vi "Accurate Measure With Setting.vi"(0 "DMM ref in":refnum<visa-resource-name>, 1 "Accurate Measure Setting":T1={"Enable DMM Relay"=FALSE, "Measure Current Only"=FALSE, [], "channel_count"=11}, 2 "P_current_count":i32, 3 "N_current_count":i32, 5 "DMM error in":errorcluster, 7 "Current Sense \nResitance Array":dbl[](array[numeric])=[1.0032214, 1.00250644, 1.00234822, 1.0040944, 1.0017711, 1.00229431, 1.00344206, 1.00482066, 1.00381056, 1.00290978, 1.00333016, 1.00367587], 9 "ESP32 ref in":refnum<visa-resource-name>, 11 "ESP32 error in":errorcluster, 12 "current_mode":u8[](array[numeric])=[0, 0, 0, 0, 0, 0, 0, 0, 0, 0, 0]) -> (4 "DMM ref out":refnum<visa-resource-name>, 6 "DMM error out":errorcluster, 8 "Accurate Data":dbl[](array[numeric]), 10 "ESP32 ref out":refnum<visa-resource-name>, 13 "time_out_count":i32, 14 "Standard Deviation of Data":dbl[](array[numeric]), 15 "ESP32 error out":errorcluster)   [LabVIEW 2023]
uses:
  <instrlib>/Agilent 3446X Series/Agilent 3446X Series.lvlib
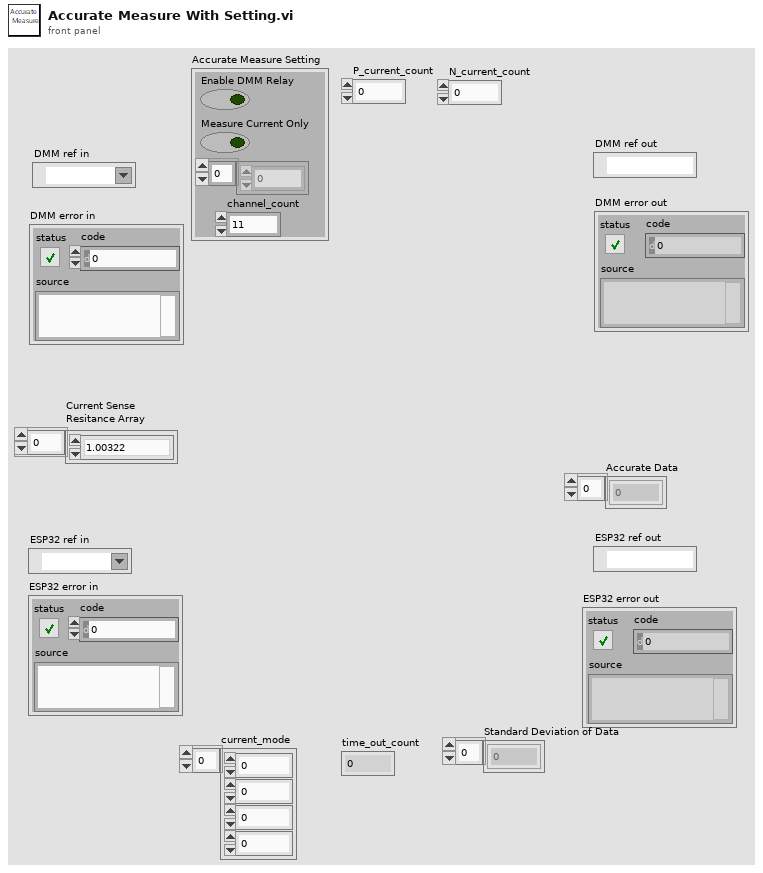
[diagram p1: front panel]
types:
  T1 = cluster{"Enable DMM Relay":bool, "Measure Current Only":bool, dbl[], "channel_count":i32}
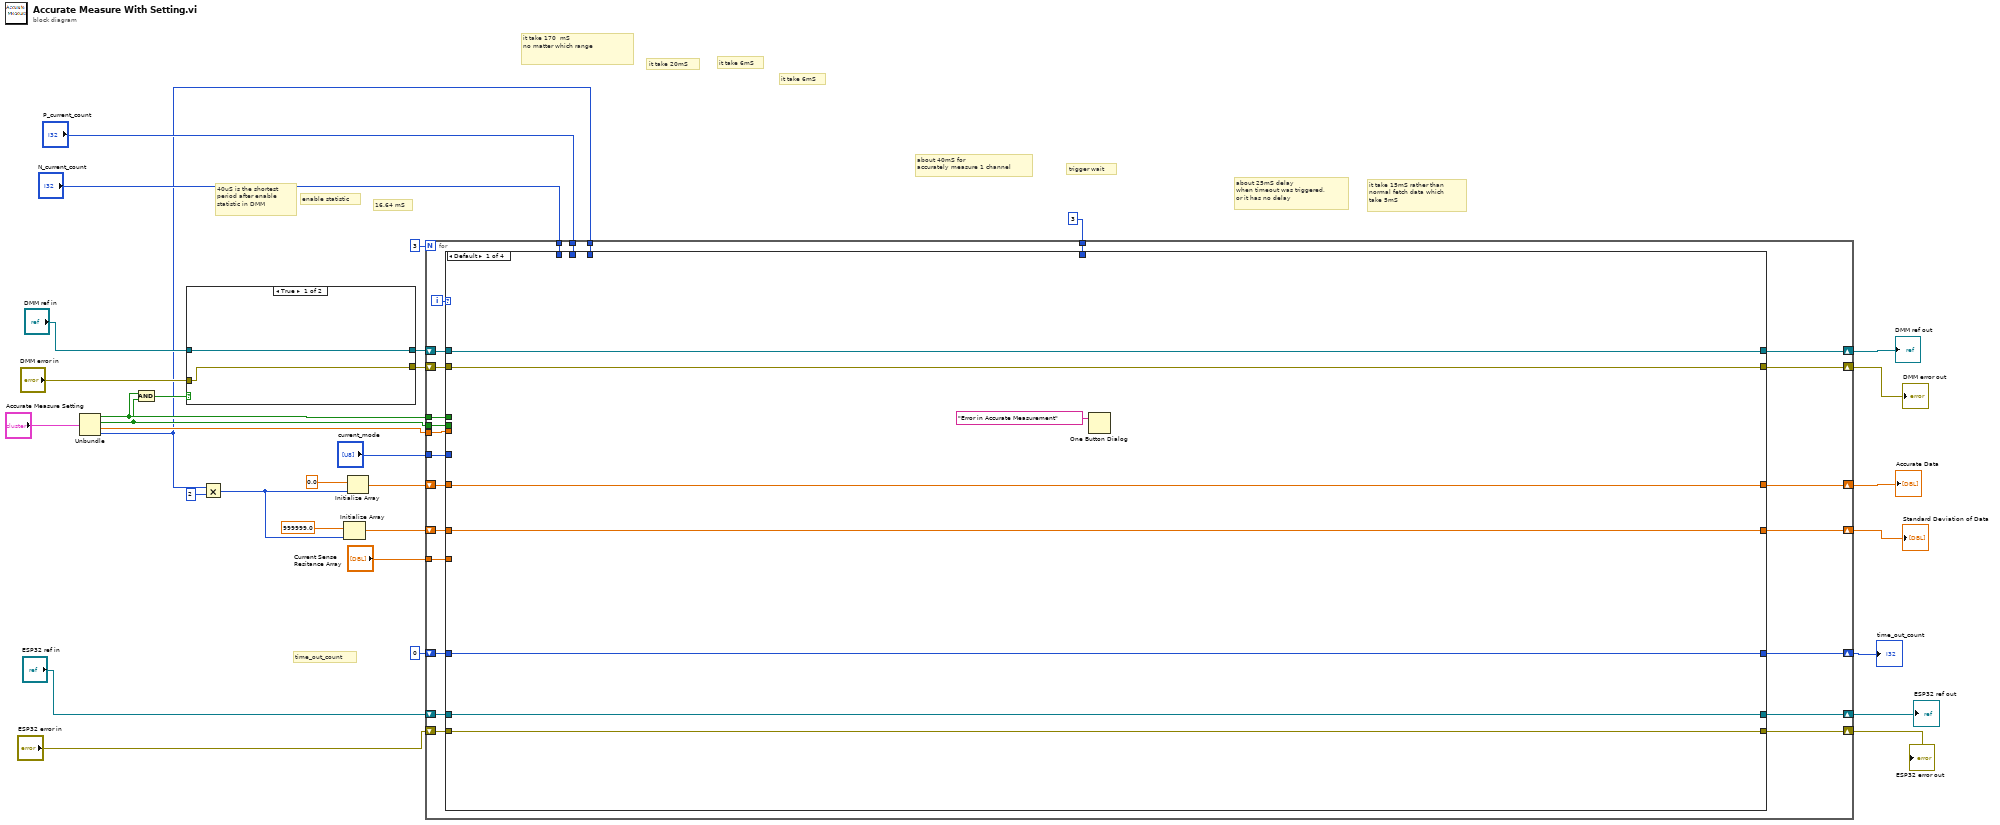
[diagram p0: block diagram]
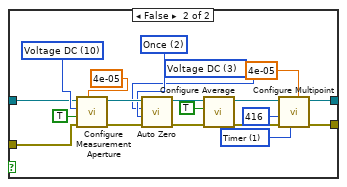
[diagram p2: hidden frame]
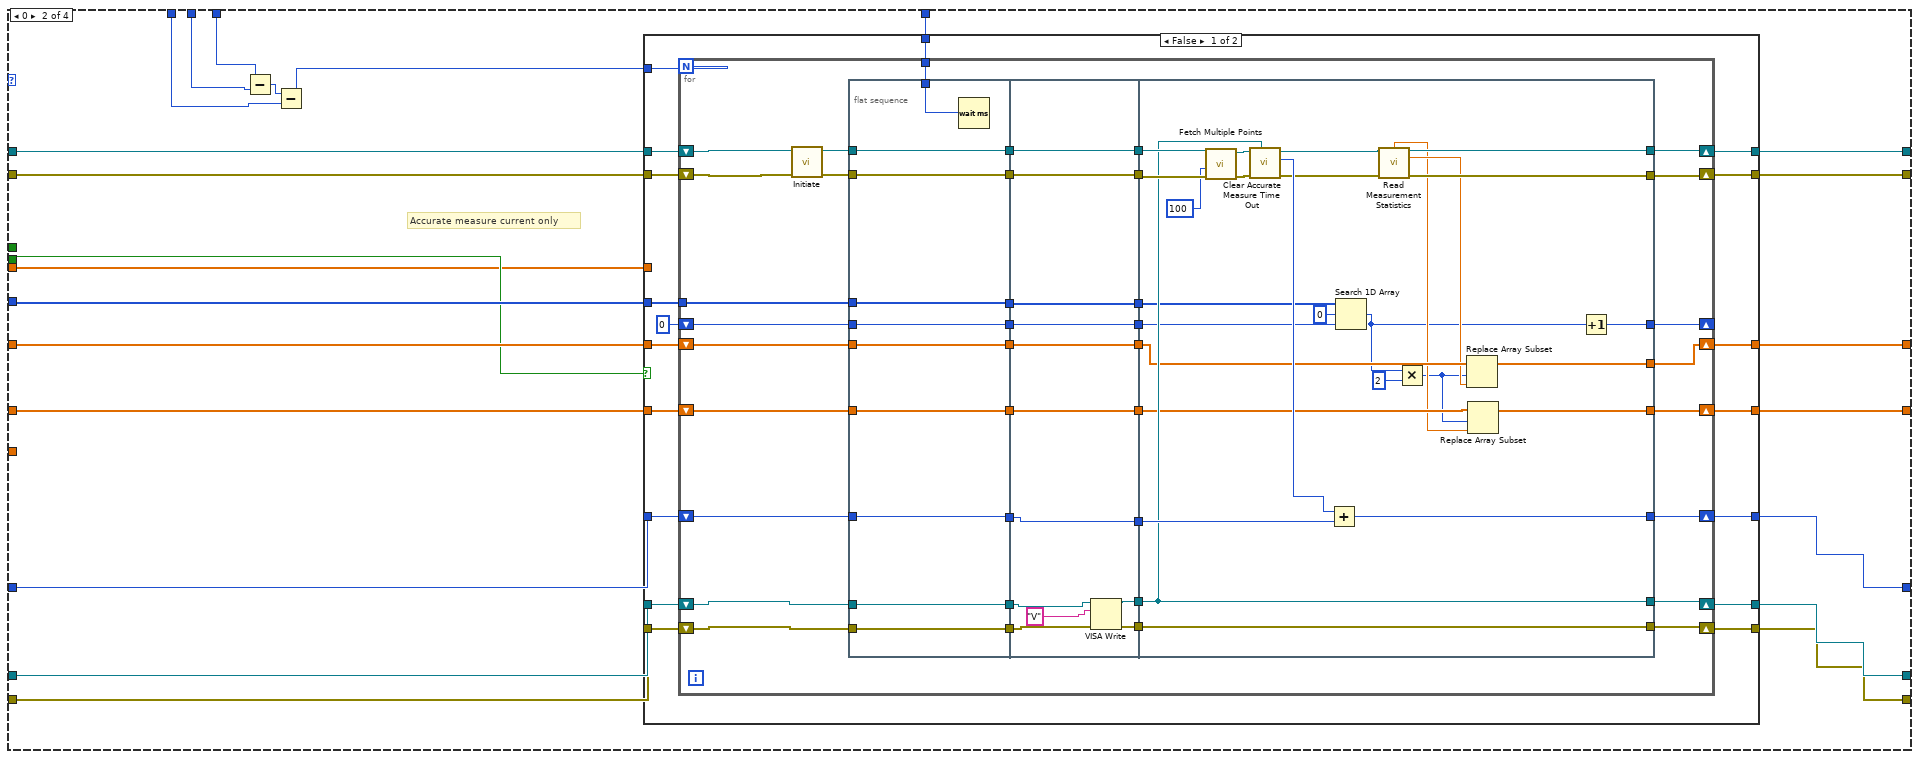
[diagram p3: hidden frame]
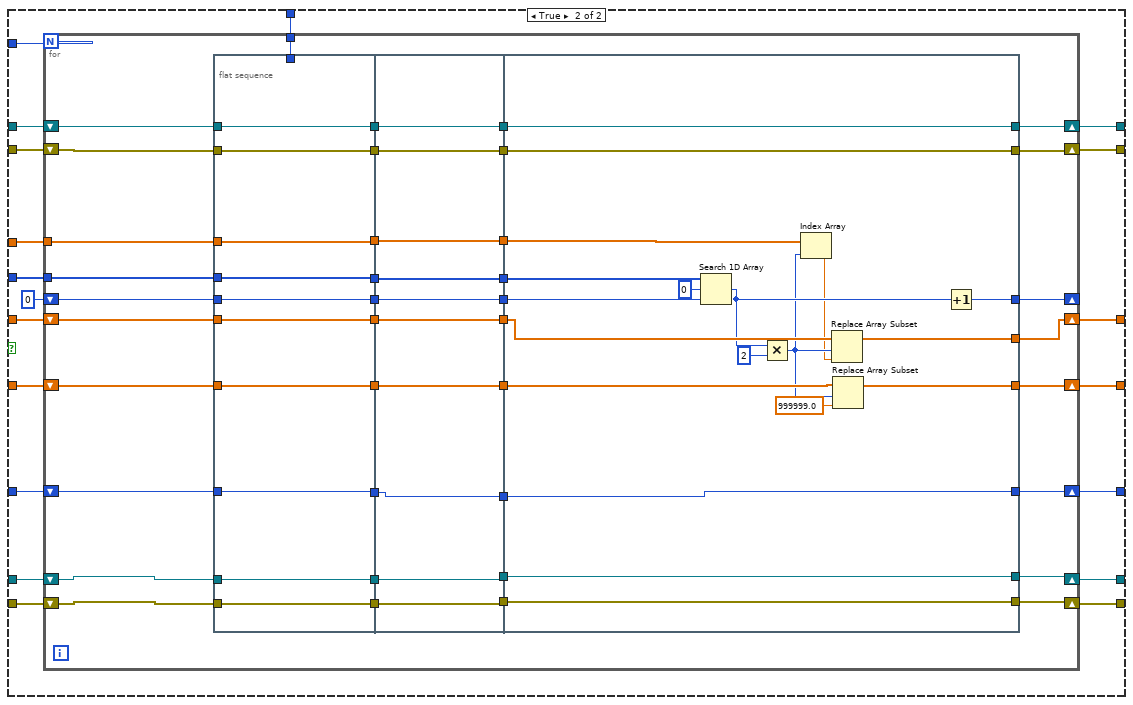
[diagram p4: hidden frame]
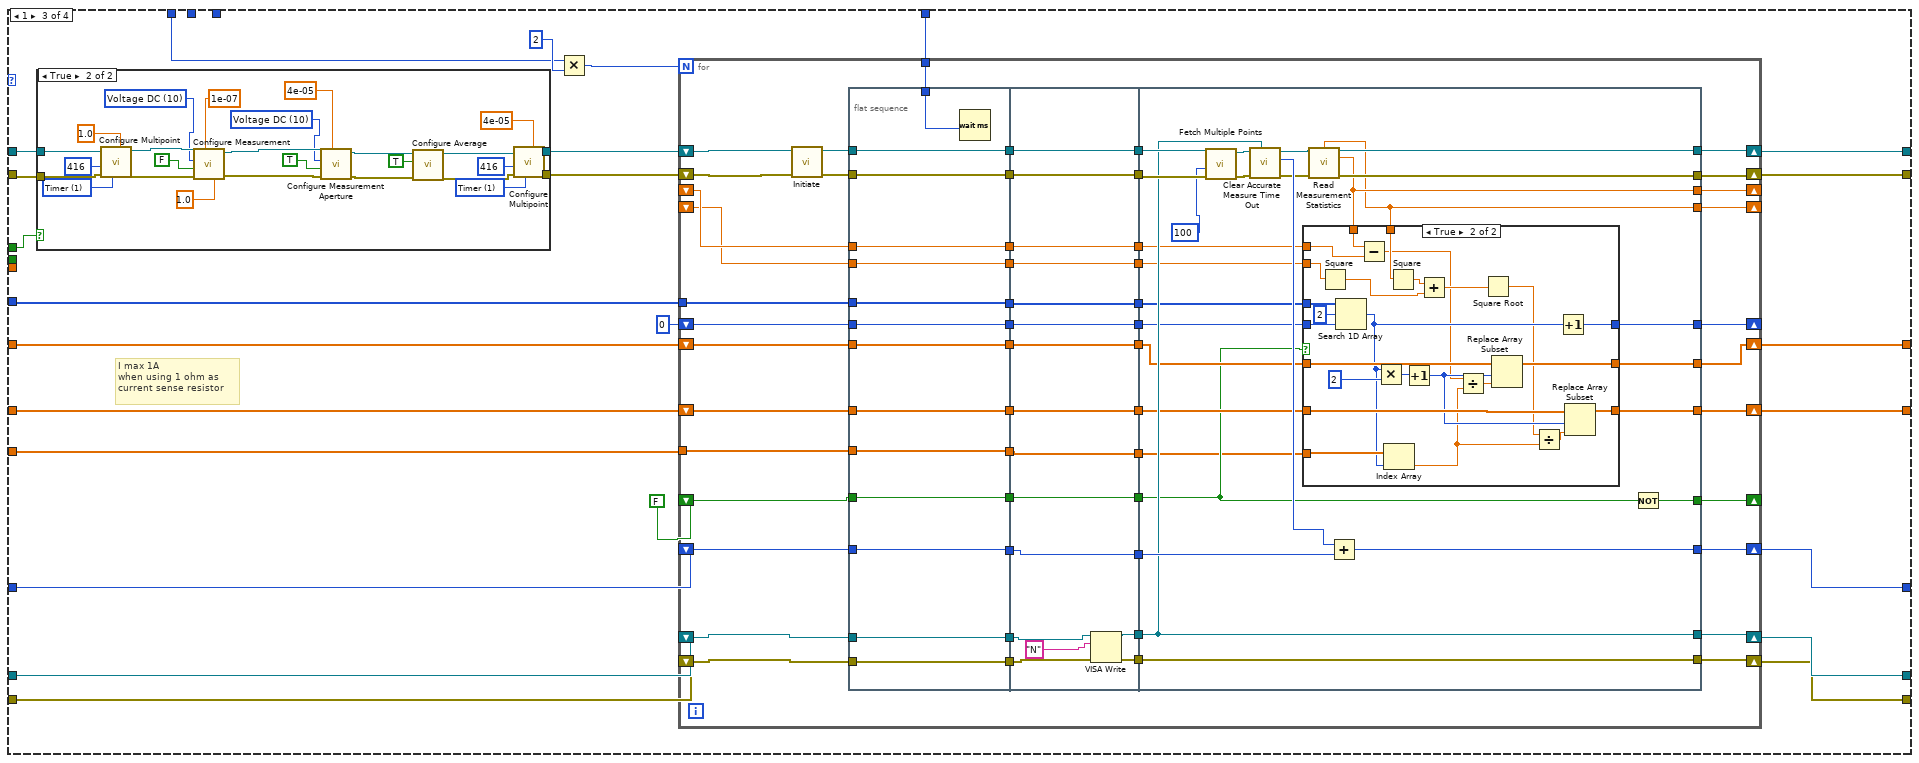
[diagram p5: hidden frame]
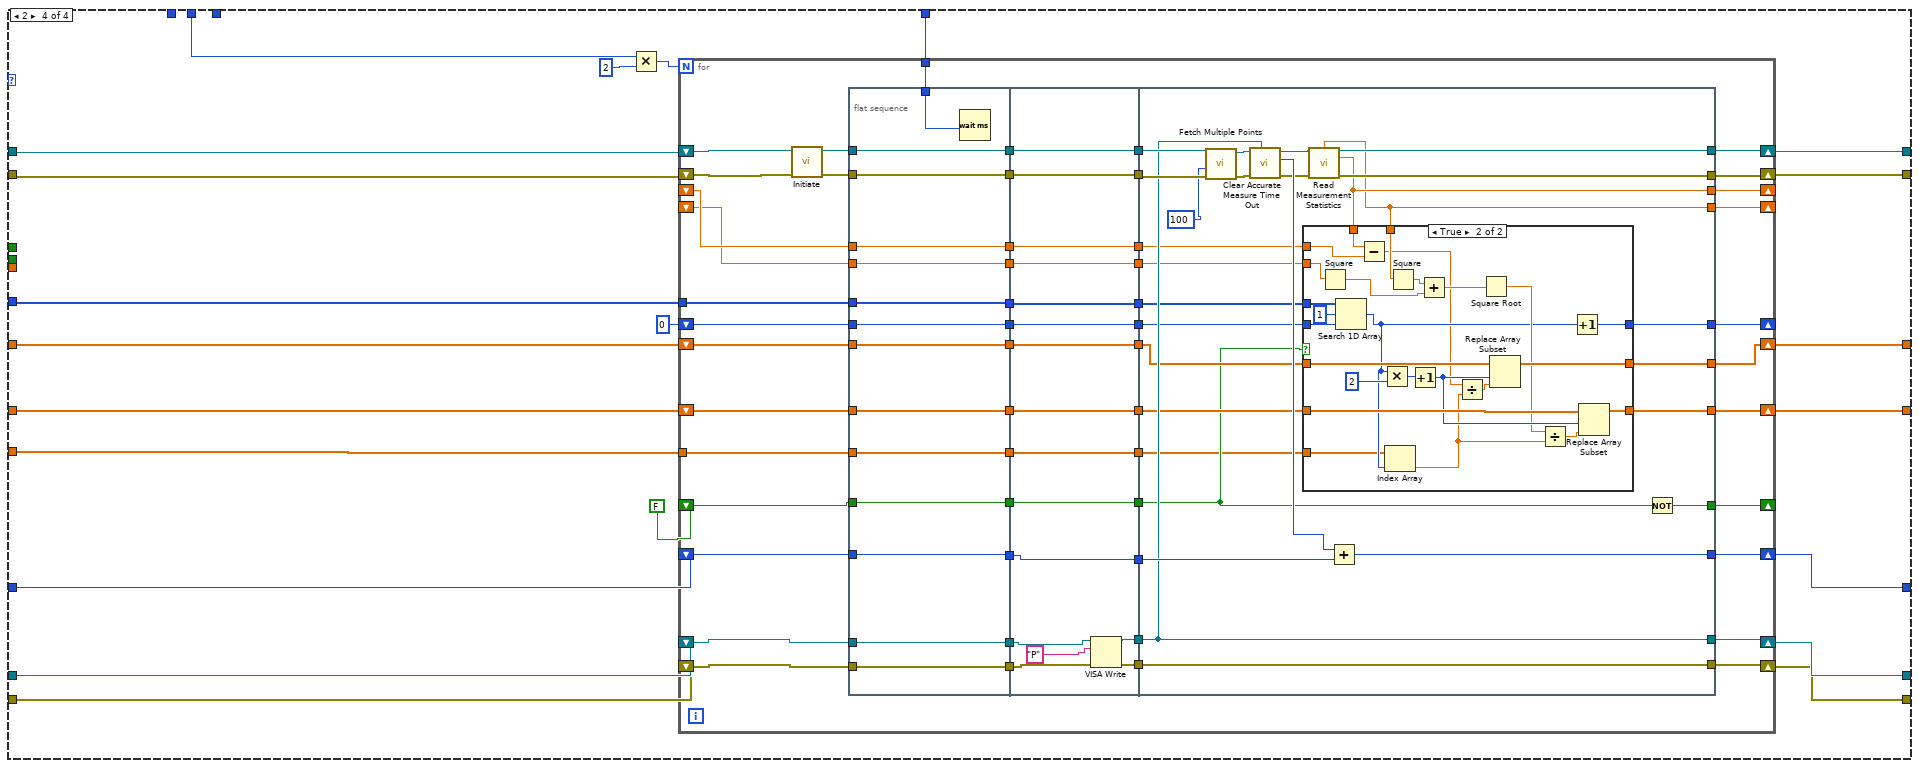
[diagram p8: hidden frame]
diagram:
  # "it take 6mS"
  # "it take 6mS"
  # "it take 20mS"
  # "it take 170  mS\nno matter which range"
  # "it take 15mS rather than\nnormal fetch data which \ntake 5mS"
  # "about 40mS for \naccurately measure 1 channel"
  # "about 25mS delay\nwhen timeout was triggered,\nor it has no delay"
  # "time_out_count"
  # "trigger wait"
  # "16.64 mS"
  # "enable statistic"
  # "40uS is the shortest\nperiod after enable \nstatistic in DMM"
  n1 = Unbundle("Accurate Measure Setting") -> ("Enable DMM Relay"=w5:bool, "Measure Current Only"=w4:bool, w6:dbl[], "channel_count"=w2:i32)
  n2 = And(x=w5, y=w4) -> (x .and. y?=w3:bool)
  n3 = case shown="True" w3 {
    tunnel: [w34 w38] -> w32
    tunnel: [w33 w37] -> w31
    tunnel: "DMM ref in" -> [w34 w36]
    tunnel: "DMM error in" -> [w33 w35]
    frame True {
    }
    frame False {
      w40 = 1 items=["Immediate", "Timer"] ("Sample Source (0: Immediate)")
      w47 = 3 items=["Current DC", "Resistance", "Temperature", "Voltage DC"] ("Zero Type (0: Current DC)")
      w48 = 2 items=["Disable", "Enable", "Once"] ("Auto Zero (1: Enable)")
      w44 = 10 items=["Continuity", "Current AC", "Current DC", "Diode", "Frequency", "Resistance 4-wire", "Period", "Resistance 2-wire", "Temperature", "Voltage AC", "Voltage DC", "Voltage DC Ratio", "Capacitance"] ("Measurement Function (0: Continuity)")
      n4 = call <instrlib>:"Configure Measurement Aperture.vi"("Aperture Time (0.1s)"=4e-05, "error in (no error)"=w35, "Enable Aperture (F: Disable)"=TRUE, "Measurement Function (0: Continuity)"=w44, "VISA resource name"=w36) -> ("error out"=w51:errorcluster, "VISA resource name out"=w50:refnum<visa-resource-name>)  [unwired: 5 in]
      n5 = call <instrlib>:"Auto Zero.vi"("error in (no error)"=w51, "Auto Zero (1: Enable)"=w48, "Zero Type (0: Current DC)"=w47, "VISA resource name"=w50) -> ("error out"=w53:errorcluster, "VISA resource name out"=w52:refnum<visa-resource-name>)  [unwired: 6 in]
      n6 = call <instrlib>:"Configure Average.vi"("error in (no error)"=w53, "Enable Statistics (F: Disable)"=TRUE, "VISA resource name"=w52) -> ("error out"=w42:errorcluster, "VISA resource name out"=w43:refnum<visa-resource-name>)  [unwired: 7 in]
      n7 = call <instrlib>:"Configure Multipoint.vi"("Sample Interval (1 Second)"=4e-05, "Sample Source (0: Immediate)"=w40, "error in (no error)"=w42, "Sample Count (1)"=416, "VISA resource name"=w43) -> ("error out"=w37:errorcluster, "VISA resource name out"=w38:refnum<visa-resource-name>)  [unwired: 2 in, 3 out]
    }
  }
  n8 = Multiply(x=w2, y=2) -> (x*y=w8:i32)
  n9 = Initialize Array(999999.0 ("Arithmetic Mean"), w8) -> (w17:dbl[])
  n10 = Initialize Array(0.0 ("Arithmetic Mean"), w8) -> (w20:dbl[])
  n11 = for {
    N: 3 -> [_]
    shift-right: [w75] -> w13
    shift-left: "ESP32 ref in" -> [w77]
    shift-right: [w74] -> w12
    shift-left: "ESP32 error in" -> [w76]
    shift-right: [w71] -> w15
    shift-left: w32 -> [w73]
    shift-right: [w70] -> w14
    shift-left: w31 -> [w72]
    tunnel: w2 -> [w69]
    tunnel: "P_current_count" -> [w68]
    tunnel: "N_current_count" -> [w67]
    tunnel: u32 3 ("milliseconds to wait") -> [w66]
    shift-right: [w65] -> w22
    shift-left: 0 -> [w64]
    shift-right: [w58] -> w11
    shift-left: w20 -> [w63]
    tunnel: "current_mode" -> [w62]
    shift-right: [w59] -> w10
    shift-left: w17 -> [w60]
    tunnel: w5 -> [w57]
    tunnel: w4 -> [w56]
    tunnel: w6 -> [w55]
    tunnel: "Current Sense \nResitance Array" -> [w54]
    i -> [w61]
    n12 = case shown="Default" w61 {
      tunnel: w77 -> [w83 w104 w335 w524]
      tunnel: w76 -> [w82 w103 w334 w523]
      tunnel: [w83 w100 w331 w520] -> w75
      tunnel: [w82 w99 w330 w519] -> w74
      tunnel: w73 -> [w85 w106 w319 w505]
      tunnel: w72 -> [w84 w105 w318 w504]
      tunnel: [w85 w102 w333 w522] -> w71
      tunnel: [w84 w101 w332 w521] -> w70
      tunnel: w69 -> [_ w98 _ _]
      tunnel: w68 -> [_ w97 _ w507]
      tunnel: w67 -> [_ w96 w314 _]
      tunnel: [w79 w94 w328 w517] -> w65
      tunnel: w66 -> [_ w95 w329 w518]
      tunnel: w64 -> [w79 w93 w327 w516]
      tunnel: w63 -> [w81 w91 w325 w514]
      tunnel: w62 -> [_ w92 w326 w515]
      tunnel: w60 -> [w80 w90 w323 w512]
      tunnel: [w80 w89 w322 w511] -> w59
      tunnel: [w81 w88 w321 w510] -> w58
      tunnel: w57 -> [_ _ w312 _]
      tunnel: w56 -> [_ w87 _ _]
      tunnel: w55 -> [_ w86 _ _]
      tunnel: w54 -> [_ _ w311 w503]
      frame Default {
        n13 = One Button Dialog(message="Error in Accurate Measurement") -> ()  [unwired: 1 in, 1 out]
      }
      frame 0 {
        # "Accurate measure current only"
        n14 = Subtract(x=w98, y=w97) -> (x-y=w108:i32)
        n15 = Subtract(x=w108, y=w96) -> (x-y=w107:i32)
        n16 = case shown="False" w87 {
          tunnel: w107 -> [w126 w232]
          tunnel: w106 -> [w125 w231]
          tunnel: w105 -> [w124 w230]
          tunnel: w104 -> [w123 w229]
          tunnel: w103 -> [w122 w228]
          tunnel: [w121 w227] -> w102
          tunnel: [w120 w226] -> w101
          tunnel: [w119 w225] -> w100
          tunnel: [w118 w224] -> w99
          tunnel: w95 -> [w117 w223]
          tunnel: [w116 w222] -> w94
          tunnel: w93 -> [w115 w221]
          tunnel: w92 -> [w114 w220]
          tunnel: w91 -> [w113 w219]
          tunnel: w90 -> [w111 w217]
          tunnel: [w110 w216] -> w89
          tunnel: [w109 w215] -> w88
          tunnel: w86 -> [_ w214]
          frame False {
            n17 = for {
              N: w126 -> [_]
              shift-right: [w160] -> w121
              shift-left: w125 -> [w164]
              shift-right: [w159] -> w120
              shift-left: w124 -> [w163]
              shift-right: [w158] -> w119
              shift-left: w123 -> [w162]
              shift-right: [w157] -> w118
              shift-left: w122 -> [w161]
              tunnel: w117 -> [w143]
              shift-right: [w142] -> w116
              shift-left: w115 -> [w156]
              tunnel: w114 -> [w140]
              shift-right: [w128] -> w109
              shift-left: w113 -> [w137]
              shift-right: [w132] -> _
              shift-left: 0 ("index of element") -> [w133]
              shift-right: [w127] -> w110
              shift-left: w111 -> [w130]
              n18 = call <instrlib>:"Initiate.vi"("error in (no error)"=w163, "VISA resource name"=w164) -> ("error out"=w144:errorcluster, "VISA resource name out"=w145:refnum<visa-resource-name>)  [unwired: 8 in]
              n19 = flat-sequence {
                tunnel: [w174] -> w155
                tunnel: w162 -> [w174]
                tunnel: [w173] -> w154
                tunnel: w161 -> [w173]
                tunnel: w145 -> [w172]
                tunnel: [w172] -> w153
                tunnel: [w171] -> w152
                tunnel: w144 -> [w171]
                tunnel: [w170] -> w151
                tunnel: w156 -> [w170]
                tunnel: w143 -> [w169]
                tunnel: [w168] -> w141
                tunnel: w140 -> [w168]
                tunnel: [w167] -> w138
                tunnel: w137 -> [w167]
                tunnel: w133 -> [w166]
                tunnel: [w166] -> w135
                tunnel: [w165] -> w131
                tunnel: w130 -> [w165]
                tunnel: w155 -> [w186]
                tunnel: w154 -> [w185]
                tunnel: w153 -> [w184]
                tunnel: [w184] -> w147
                tunnel: w152 -> [w183]
                tunnel: [w183] -> w148
                tunnel: [w182] -> w149
                tunnel: [w181] -> w150
                tunnel: w151 -> [w179]
                tunnel: [w179] -> w146
                tunnel: w141 -> [w178]
                tunnel: [w178] -> w139
                tunnel: w138 -> [w177]
                tunnel: [w177] -> w136
                tunnel: w135 -> [w176]
                tunnel: [w176] -> w134
                tunnel: w131 -> [w175]
                tunnel: [w175] -> w129
                tunnel: [w213] -> w157
                tunnel: [w201] -> w158
                tunnel: [w205] -> w159
                tunnel: [w206] -> w160
                tunnel: w150 -> [w213]
                tunnel: w149 -> [w201]
                tunnel: w148 -> [w212]
                tunnel: w147 -> [w211]
                tunnel: [w207] -> w142
                tunnel: w146 -> [w202]
                tunnel: w139 -> [w200]
                tunnel: w136 -> [w196]
                tunnel: w134 -> [w198]
                tunnel: [w197] -> w132
                tunnel: w129 -> [w194]
                tunnel: [w192] -> w128
                tunnel: [w191] -> w127
                frame #0 {
                  n20 = Wait (ms)(milliseconds to wait=w169) -> ()  [unwired: 1 out]
                }
                frame #1 {
                  n21 = VISA Write(VISA resource name=w186, write buffer="V" ("data in"), error in (no error)=w185) -> (VISA resource name out=w182:refnum<visa-resource-name>, error out=w181:errorcluster)  [unwired: 1 out]
                }
                frame #2 {
                  n22 = call <instrlib>:"Fetch Multiple Points.vi"("error in (no error)"=w212, "Timeout (10000 ms)"=100, "VISA resource name"=w211) -> ("error out"=w209:errorcluster, "VISA resource name out"=w210:refnum<visa-resource-name>)  [unwired: 1 in, 6 out]
                  n23 = call "Clear Accurate Measure Time Out.vi"("ESP32 ref"=w201, "error in (no error)"=w209, "DMM ref"=w210) -> ("error out"=w203:errorcluster, "Time out count"=w208:i32, "VISA Refnum out"=w204:refnum<visa-resource-name>)  [unwired: 5 in, 1 out]
                  n24 = Add(x=w208, y=w202) -> (x+y=w207:i32)
                  n25 = Search 1D Array(1D array=w200, element=u8 0, start index (0)=w198) -> (index of element=w189:i32)
                  n26 = call <instrlib>:"Read Measurement Statistics.vi"("VISA resource name"=w204, "error in (no error)"=w203) -> ("Standard Deviation"=w193:dbl, "VISA resource name out"=w206:refnum<visa-resource-name>, "Arithmetic Mean"=w195:dbl, "error out"=w205:errorcluster)  [unwired: 6 in, 4 out]
                  n27 = Multiply(x=w189, y=2) -> (x*y=w187:i32)
                  n28 = Replace Array Subset(array=w196, new element=w195, index=w187) -> (w192:dbl[])
                  n29 = Replace Array Subset(array=w194, new element=w193, index=w187) -> (w191:dbl[])
                  n30 = Increment(x=w189) -> (x+1=w197:i32)
                }
              }
            }
          }
          frame True {
            n31 = for {
              N: w232 -> [_]
              shift-right: [w241] -> w227
              shift-left: w231 -> [w243]
              shift-right: [w236] -> w226
              shift-left: w230 -> [w238]
              shift-right: [w269] -> w225
              shift-left: w229 -> [w271]
              shift-right: [w268] -> w224
              shift-left: w228 -> [w270]
              tunnel: w223 -> [w260]
              shift-right: [w259] -> w222
              shift-left: w221 -> [w267]
              tunnel: w220 -> [w257]
              shift-right: [w245] -> w215
              shift-left: w219 -> [w254]
              shift-right: [w249] -> _
              shift-left: 0 ("index of element") -> [w250]
              shift-right: [w244] -> w216
              shift-left: w217 -> [w247]
              tunnel: w214 -> [w233]
              n32 = flat-sequence {
                tunnel: [w281] -> w266
                tunnel: w271 -> [w281]
                tunnel: [w280] -> w265
                tunnel: w270 -> [w280]
                tunnel: [w279] -> w264
                tunnel: w267 -> [w279]
                tunnel: w260 -> [_]
                tunnel: [w278] -> w258
                tunnel: w257 -> [w278]
                tunnel: [w277] -> w255
                tunnel: w254 -> [w277]
                tunnel: w250 -> [w276]
                tunnel: [w276] -> w252
                tunnel: [w275] -> w248
                tunnel: w247 -> [w275]
                tunnel: w243 -> [w274]
                tunnel: [w274] -> w240
                tunnel: [w273] -> w239
                tunnel: w238 -> [w273]
                tunnel: [w272] -> w235
                tunnel: w233 -> [w272]
                tunnel: w266 -> [w284]
                tunnel: w265 -> [w283]
                tunnel: [w284] -> w262
                tunnel: [w283] -> w263
                tunnel: w264 -> [w291]
                tunnel: [w291] -> w261
                tunnel: w258 -> [w290]
                tunnel: [w290] -> w256
                tunnel: w255 -> [w289]
                tunnel: [w289] -> w253
                tunnel: w252 -> [w288]
                tunnel: [w288] -> w251
                tunnel: w248 -> [w287]
                tunnel: [w287] -> w246
                tunnel: [w286] -> w242
                tunnel: w240 -> [w286]
                tunnel: w239 -> [w285]
                tunnel: [w285] -> w237
                tunnel: w235 -> [w282]
                tunnel: [w282] -> w234
                tunnel: [w310] -> w268
                tunnel: [w309] -> w269
                tunnel: w263 -> [w310]
                tunnel: w262 -> [w309]
                tunnel: [w292] -> w259
                tunnel: w261 -> [w292]
                tunnel: w256 -> [w308]
                tunnel: w253 -> [w304]
                tunnel: w251 -> [w306]
                tunnel: [w305] -> w249
                tunnel: w246 -> [w303]
                tunnel: [w302] -> w245
                tunnel: [w301] -> w244
                tunnel: w242 -> [w298]
                tunnel: [w298] -> w241
                tunnel: [w297] -> w236
                tunnel: w237 -> [w297]
                tunnel: w234 -> [w295]
                frame #0 {
                }
                frame #1 {
                }
                frame #2 {
                  n33 = Search 1D Array(1D array=w308, element=u8 0, start index (0)=w306) -> (index of element=w300:i32)
                  n34 = Multiply(x=w300, y=2) -> (x*y=w294:i32)
                  n35 = Index Array(array=w295, index=w294) -> (element=w293:dbl)
                  n36 = Replace Array Subset(array=w304, new element=w293, index=w294) -> (w302:dbl[])
                  n37 = Replace Array Subset(array=w303, new element=999999.0 ("new element/subarray"), index=w294) -> (w301:dbl[])
                  n38 = Increment(x=w300) -> (x+1=w305:i32)
                }
              }
            }
          }
        }
      }
      frame 1 {
        # "I max 1A\nwhen using 1 ohm as \ncurrent sense resistor"
        n39 = case shown="True" w312 {
          tunnel: w319 -> [w337 w343]
          tunnel: w318 -> [w336 w342]
          tunnel: [w337 w341] -> w317
          tunnel: [w336 w340] -> w316
          frame False {
          }
          frame True {
            w353 = 1 items=["Immediate", "Timer"] ("Sample Source (0: Immediate)")
            w349 = 10 items=["Continuity", "Current AC", "Current DC", "Diode", "Frequency", "Resistance 4-wire", "Period", "Resistance 2-wire", "Temperature", "Voltage AC", "Voltage DC", "Voltage DC Ratio", "Capacitance"] ("Measurement Function (0: Continuity)")
            w347 = 1 items=["Immediate", "Timer"] ("Sample Source (0: Immediate)")
            w344 = 10 items=["Continuity", "Current AC", "Current DC", "Diode", "Frequency", "Resistance 4-wire", "Period", "Resistance 2-wire", "Temperature", "Voltage AC", "Voltage DC", "Voltage DC Ratio", "Capacitance"] ("Measurement Function (10: Voltage DC)")
            n40 = call <instrlib>:"Configure Multipoint.vi"("Sample Interval (1 Second)"=1.0, "Sample Source (0: Immediate)"=w347, "error in (no error)"=w342, "Sample Count (1)"=416, "VISA resource name"=w343) -> ("error out"=w360:errorcluster, "VISA resource name out"=w359:refnum<visa-resource-name>)  [unwired: 2 in, 3 out]
            n41 = call <instrlib>:"Configure Measurement.vi"("Manual Range (1)"=1.0, "Absolute Resolution (1E-6)"=1e-07 ("x"), "error in (no error)"=w360, "Auto Range (T: Enable)"=FALSE, "Measurement Function (10: Voltage DC)"=w344, "VISA resource name"=w359) -> ("error out"=w357:errorcluster, "VISA resource name out"=w358:refnum<visa-resource-name>)  [unwired: 4 out]
            n42 = call <instrlib>:"Configure Measurement Aperture.vi"("Aperture Time (0.1s)"=4e-05, "error in (no error)"=w357, "Enable Aperture (F: Disable)"=TRUE, "Measurement Function (0: Continuity)"=w349, "VISA resource name"=w358) -> ("error out"=w362:errorcluster, "VISA resource name out"=w363:refnum<visa-resource-name>)  [unwired: 5 in]
            n43 = call <instrlib>:"Configure Average.vi"("error in (no error)"=w362, "Enable Statistics (F: Disable)"=TRUE, "VISA resource name"=w363) -> ("error out"=w361:errorcluster, "VISA resource name out"=w356:refnum<visa-resource-name>)  [unwired: 7 in]
            n44 = call <instrlib>:"Configure Multipoint.vi"("Sample Interval (1 Second)"=4e-05, "Sample Source (0: Immediate)"=w353, "error in (no error)"=w361, "Sample Count (1)"=416, "VISA resource name"=w356) -> ("error out"=w340:errorcluster, "VISA resource name out"=w341:refnum<visa-resource-name>)  [unwired: 2 in, 3 out]
          }
        }
        n45 = Multiply(x=w314, y=2) -> (x*y=w315:i32)
        n46 = for {
          N: w315 -> [_]
          shift-right: [w412] -> w333
          shift-left: w317 -> [w416]
          shift-right: [w411] -> w332
          shift-left: w316 -> [w415]
          shift-right: [w410] -> w331
          shift-left: w335 -> [w414]
          shift-right: [w409] -> w330
          shift-left: w334 -> [w413]
          tunnel: w329 -> [w395]
          shift-right: [w394] -> w328
          shift-left: w327 -> [w408]
          tunnel: w326 -> [w392]
          shift-right: [w380] -> w321
          shift-left: w325 -> [w389]
          shift-right: [w384] -> _
          shift-left: 0 ("index of element") -> [w385]
          shift-right: [w379] -> w322
          shift-left: w323 -> [w382]
          shift-right: [w375] -> _
          shift-left: FALSE ("Enable Statistics (F: Disable)") -> [w376]
          shift-right: [w374] -> _
          shift-left: _ -> [w372]
          shift-right: [w373] -> _
          shift-left: _ -> [w369]
          tunnel: w311 -> [w365]
          n47 = call <instrlib>:"Initiate.vi"("error in (no error)"=w415, "VISA resource name"=w416) -> ("error out"=w396:errorcluster, "VISA resource name out"=w397:refnum<visa-resource-name>)  [unwired: 8 in]
          n48 = flat-sequence {
            tunnel: [w430] -> w407
            tunnel: w414 -> [w430]
            tunnel: [w429] -> w406
            tunnel: w413 -> [w429]
            tunnel: w397 -> [w428]
            tunnel: [w428] -> w405
            tunnel: [w427] -> w404
            tunnel: w396 -> [w427]
            tunnel: [w426] -> w403
            tunnel: w408 -> [w426]
            tunnel: w395 -> [w425]
            tunnel: [w424] -> w393
            tunnel: w392 -> [w424]
            tunnel: [w423] -> w390
            tunnel: w389 -> [w423]
            tunnel: w385 -> [w422]
            tunnel: [w422] -> w387
            tunnel: [w421] -> w383
            tunnel: w382 -> [w421]
            tunnel: w376 -> [w420]
            tunnel: [w420] -> w378
            tunnel: w372 -> [w419]
            tunnel: [w419] -> w370
            tunnel: w369 -> [w418]
            tunnel: [w418] -> w368
            tunnel: [w417] -> w366
            tunnel: w365 -> [w417]
            tunnel: w407 -> [w446]
            tunnel: w406 -> [w445]
            tunnel: w405 -> [w444]
            tunnel: [w444] -> w399
            tunnel: w404 -> [w443]
            tunnel: [w443] -> w400
            tunnel: [w442] -> w401
            tunnel: [w441] -> w402
            tunnel: w403 -> [w439]
            tunnel: [w439] -> w398
            tunnel: w393 -> [w438]
            tunnel: [w438] -> w391
            tunnel: w390 -> [w437]
            tunnel: [w437] -> w388
            tunnel: w387 -> [w436]
            tunnel: [w436] -> w386
            tunnel: w383 -> [w435]
            tunnel: [w435] -> w381
            tunnel: w378 -> [w434]
            tunnel: [w434] -> w377
            tunnel: [w433] -> w371
            tunnel: w370 -> [w433]
            tunnel: w368 -> [w432]
            tunnel: [w432] -> w367
            tunnel: w366 -> [w431]
            tunnel: [w431] -> w364
            tunnel: [w474] -> w409
            tunnel: [w462] -> w410
            tunnel: [w466] -> w411
            tunnel: [w467] -> w412
            tunnel: w402 -> [w474]
            tunnel: w401 -> [w462]
            tunnel: w400 -> [w473]
            tunnel: w399 -> [w472]
            tunnel: [w468] -> w394
            tunnel: w398 -> [w463]
            tunnel: w391 -> [w461]
            tunnel: w388 -> [w458]
            tunnel: w386 -> [w460]
            tunnel: [w459] -> w384
            tunnel: w381 -> [w457]
            tunnel: [w456] -> w380
            tunnel: [w455] -> w379
            tunnel: w377 -> [w454]
            tunnel: [w453] -> w375
            tunnel: [w450] -> w374
            tunnel: [w449] -> w373
            tunnel: w371 -> [w452]
            tunnel: w367 -> [w451]
            tunnel: w364 -> [w447]
            frame #0 {
              n49 = Wait (ms)(milliseconds to wait=w425) -> ()  [unwired: 1 out]
            }
            frame #1 {
              n50 = VISA Write(VISA resource name=w446, write buffer="N" ("data in"), error in (no error)=w445) -> (VISA resource name out=w442:refnum<visa-resource-name>, error out=w441:errorcluster)  [unwired: 1 out]
            }
            frame #2 {
              n51 = call <instrlib>:"Fetch Multiple Points.vi"("error in (no error)"=w473, "Timeout (10000 ms)"=100, "VISA resource name"=w472) -> ("error out"=w470:errorcluster, "VISA resource name out"=w471:refnum<visa-resource-name>)  [unwired: 1 in, 6 out]
              n52 = call "Clear Accurate Measure Time Out.vi"("ESP32 ref"=w462, "error in (no error)"=w470, "DMM ref"=w471) -> ("error out"=w464:errorcluster, "Time out count"=w469:i32, "VISA Refnum out"=w465:refnum<visa-resource-name>)  [unwired: 5 in, 1 out]
              n53 = call <instrlib>:"Read Measurement Statistics.vi"("VISA resource name"=w465, "error in (no error)"=w464) -> ("Standard Deviation"=w449:dbl, "VISA resource name out"=w467:refnum<visa-resource-name>, "Arithmetic Mean"=w450:dbl, "error out"=w466:errorcluster)  [unwired: 6 in, 4 out]
              n54 = case shown="True" w454 {
                tunnel: w461 -> [_ w502]
                tunnel: w460 -> [w477 w500]
                tunnel: [w477 w499] -> w459
                tunnel: w458 -> [w476 w498]
                tunnel: w457 -> [w475 w497]
                tunnel: [w476 w496] -> w456
                tunnel: [w475 w495] -> w455
                tunnel: w452 -> [_ w488]
                tunnel: w451 -> [_ w494]
                tunnel: w450 -> [_ w489]
                tunnel: w449 -> [_ w493]
                tunnel: w447 -> [_ w484]
                frame False {
                }
                frame True {
                  n55 = Square(x=w494) -> (x^2=w491:dbl)
                  n56 = Search 1D Array(1D array=w502, element=u8 2, start index (0)=w500) -> (index of element=w483:i32)
                  n57 = Subtract(x=w489, y=w488) -> (x-y=w481:dbl)
                  n58 = Multiply(x=w483, y=2) -> (x*y=w486:i32)
                  n59 = Index Array(array=w484, index=w483) -> (element=w478:dbl)
                  n60 = Square(x=w493) -> (x^2=w492:dbl)
                  n61 = Increment(x=w486) -> (x+1=w485:i32)
                  n62 = Add(x=w492, y=w491) -> (x+y=w490:dbl)
                  n63 = Divide(x=w481, y=w478) -> (x/y=w482:dbl)
                  n64 = Square Root(x=w490) -> (sqrt(x)=w479:dbl)
                  n65 = Replace Array Subset(array=w498, new element=w482, index=w485) -> (w496:dbl[])
                  n66 = Divide(x=w479, y=w478) -> (x/y=w480:dbl)
                  n67 = Increment(x=w483) -> (x+1=w499:i32)
                  n68 = Replace Array Subset(array=w497, new element=w480, index=w485) -> (w495:dbl[])
                }
              }
              n69 = Add(x=w469, y=w463) -> (x+y=w468:i32)
              n70 = Not(x=w454) -> (.not. x?=w453:bool)
            }
          }
        }
      }
      frame 2 {
        n71 = Multiply(x=w507, y=2) -> (x*y=w506:i32)
        n72 = for {
          N: w506 -> [_]
          shift-right: [w573] -> w522
          shift-left: w505 -> [w577]
          shift-right: [w572] -> w521
          shift-left: w504 -> [w576]
          shift-right: [w571] -> w520
          shift-left: w524 -> [w575]
          shift-right: [w570] -> w519
          shift-left: w523 -> [w574]
          tunnel: w518 -> [w556]
          shift-right: [w555] -> w517
          shift-left: w516 -> [w569]
          tunnel: w515 -> [w553]
          shift-right: [w541] -> w510
          shift-left: w514 -> [w550]
          shift-right: [w545] -> _
          shift-left: 0 ("index of element") -> [w546]
          shift-right: [w540] -> w511
          shift-left: w512 -> [w543]
          shift-right: [w536] -> _
          shift-left: FALSE ("Enable Statistics (F: Disable)") -> [w537]
          shift-right: [w535] -> _
          shift-left: _ -> [w533]
          shift-right: [w534] -> _
          shift-left: _ -> [w530]
          tunnel: w503 -> [w526]
          n73 = call <instrlib>:"Initiate.vi"("error in (no error)"=w576, "VISA resource name"=w577) -> ("error out"=w557:errorcluster, "VISA resource name out"=w558:refnum<visa-resource-name>)  [unwired: 8 in]
          n74 = flat-sequence {
            tunnel: [w591] -> w568
            tunnel: w575 -> [w591]
            tunnel: [w590] -> w567
            tunnel: w574 -> [w590]
            tunnel: w558 -> [w589]
            tunnel: [w589] -> w566
            tunnel: [w588] -> w565
            tunnel: w557 -> [w588]
            tunnel: [w587] -> w564
            tunnel: w569 -> [w587]
            tunnel: w556 -> [w586]
            tunnel: [w585] -> w554
            tunnel: w553 -> [w585]
            tunnel: [w584] -> w551
            tunnel: w550 -> [w584]
            tunnel: w546 -> [w583]
            tunnel: [w583] -> w548
            tunnel: [w582] -> w544
            tunnel: w543 -> [w582]
            tunnel: w537 -> [w581]
            tunnel: [w581] -> w539
            tunnel: w533 -> [w580]
            tunnel: [w580] -> w531
            tunnel: w530 -> [w579]
            tunnel: [w579] -> w529
            tunnel: [w578] -> w527
            tunnel: w526 -> [w578]
            tunnel: w568 -> [w607]
            tunnel: w567 -> [w606]
            tunnel: w566 -> [w605]
            tunnel: [w605] -> w560
            tunnel: w565 -> [w604]
            tunnel: [w604] -> w561
            tunnel: [w603] -> w562
            tunnel: [w602] -> w563
            tunnel: w564 -> [w600]
            tunnel: [w600] -> w559
            tunnel: w554 -> [w599]
            tunnel: [w599] -> w552
            tunnel: w551 -> [w598]
            tunnel: [w598] -> w549
            tunnel: w548 -> [w597]
            tunnel: [w597] -> w547
            tunnel: w544 -> [w596]
            tunnel: [w596] -> w542
            tunnel: w539 -> [w595]
            tunnel: [w595] -> w538
            tunnel: [w594] -> w532
            tunnel: w531 -> [w594]
            tunnel: w529 -> [w593]
            tunnel: [w593] -> w528
            tunnel: w527 -> [w592]
            tunnel: [w592] -> w525
            tunnel: [w635] -> w570
            tunnel: [w623] -> w571
            tunnel: [w627] -> w572
            tunnel: [w628] -> w573
            tunnel: w563 -> [w635]
            tunnel: w562 -> [w623]
            tunnel: w561 -> [w634]
            tunnel: w560 -> [w633]
            tunnel: [w629] -> w555
            tunnel: w559 -> [w624]
            tunnel: w552 -> [w622]
            tunnel: w549 -> [w619]
            tunnel: w547 -> [w621]
            tunnel: [w620] -> w545
            tunnel: w542 -> [w618]
            tunnel: [w617] -> w541
            tunnel: [w616] -> w540
            tunnel: w538 -> [w615]
            tunnel: [w614] -> w536
            tunnel: [w611] -> w535
            tunnel: [w610] -> w534
            tunnel: w532 -> [w613]
            tunnel: w528 -> [w612]
            tunnel: w525 -> [w608]
            frame #0 {
              n75 = Wait (ms)(milliseconds to wait=w586) -> ()  [unwired: 1 out]
            }
            frame #1 {
              n76 = VISA Write(VISA resource name=w607, write buffer="P" ("data in"), error in (no error)=w606) -> (VISA resource name out=w603:refnum<visa-resource-name>, error out=w602:errorcluster)  [unwired: 1 out]
            }
            frame #2 {
              n77 = call <instrlib>:"Fetch Multiple Points.vi"("error in (no error)"=w634, "Timeout (10000 ms)"=100, "VISA resource name"=w633) -> ("error out"=w631:errorcluster, "VISA resource name out"=w632:refnum<visa-resource-name>)  [unwired: 1 in, 6 out]
              n78 = call "Clear Accurate Measure Time Out.vi"("ESP32 ref"=w623, "error in (no error)"=w631, "DMM ref"=w632) -> ("error out"=w625:errorcluster, "Time out count"=w630:i32, "VISA Refnum out"=w626:refnum<visa-resource-name>)  [unwired: 5 in, 1 out]
              n79 = call <instrlib>:"Read Measurement Statistics.vi"("VISA resource name"=w626, "error in (no error)"=w625) -> ("Standard Deviation"=w610:dbl, "VISA resource name out"=w628:refnum<visa-resource-name>, "Arithmetic Mean"=w611:dbl, "error out"=w627:errorcluster)  [unwired: 6 in, 4 out]
              n80 = case shown="True" w615 {
                tunnel: w622 -> [_ w663]
                tunnel: w621 -> [w638 w661]
                tunnel: [w638 w660] -> w620
                tunnel: w619 -> [w637 w659]
                tunnel: w618 -> [w636 w658]
                tunnel: [w637 w657] -> w617
                tunnel: [w636 w656] -> w616
                tunnel: w613 -> [_ w649]
                tunnel: w612 -> [_ w655]
                tunnel: w611 -> [_ w650]
                tunnel: w610 -> [_ w654]
                tunnel: w608 -> [_ w642]
                frame False {
                }
                frame True {
                  n81 = Square(x=w655) -> (x^2=w652:dbl)
                  n82 = Search 1D Array(1D array=w663, element=u8 1, start index (0)=w661) -> (index of element=w643:i32)
                  n83 = Subtract(x=w650, y=w649) -> (x-y=w640:dbl)
                  n84 = Multiply(x=w643, y=2) -> (x*y=w647:i32)
                  n85 = Index Array(array=w642, index=w643) -> (element=w639:dbl)
                  n86 = Square(x=w654) -> (x^2=w653:dbl)
                  n87 = Increment(x=w647) -> (x+1=w646:i32)
                  n88 = Add(x=w653, y=w652) -> (x+y=w651:dbl)
                  n89 = Divide(x=w640, y=w639) -> (x/y=w641:dbl)
                  n90 = Square Root(x=w651) -> (sqrt(x)=w644:dbl)
                  n91 = Replace Array Subset(array=w659, new element=w641, index=w646) -> (w657:dbl[])
                  n92 = Divide(x=w644, y=w639) -> (x/y=w645:dbl)
                  n93 = Increment(x=w643) -> (x+1=w660:i32)
                  n94 = Replace Array Subset(array=w658, new element=w645, index=w646) -> (w656:dbl[])
                }
              }
              n95 = Add(x=w630, y=w624) -> (x+y=w629:i32)
              n96 = Not(x=w615) -> (.not. x?=w614:bool)
            }
          }
        }
      }
    }
  }
  "time_out_count" <- w22
  "DMM ref out" <- w15
  "DMM error out" <- w14
  "ESP32 ref out" <- w13
  "ESP32 error out" <- w12
  "Accurate Data" <- w11
  "Standard Deviation of Data" <- w10
